vi "borrowDataDescriptorInterface.vi"(8 "error in (no error)":errorcluster, 11 "IBaseObject in":refnum<class "IBaseObject.lvclass">) -> (0 "error out":errorcluster, 2 "DataDescriptor out":refnum<class "IDataDescriptor.lvclass">, 3 "IBaseObject out":refnum<class "IBaseObject.lvclass">)   [LabVIEW 2022 SP3, in "openDAQ.lvlib" / "IBaseObject.lvlib" / "IBaseObject.lvclass"]
uses:
  <instrlib>/openDAQ/Public/Classes/IBaseObject/IBaseObject.lvclass
  <instrlib>/openDAQ/Public/Classes/IDataDescriptor/IDataDescriptor.lvclass
  C:/Program Files (x86)/National Instruments/LabVIEW 2022/instr.lib/openDAQ/Public/Classes/IBaseObject/IBaseObject.lvclass
  <instrlib>/openDAQ/Public/Classes/IBaseObject/IBaseObject.lvclass/IBaseObject.ctl
  <instrlib>/openDAQ/Public/Classes/IBaseObject/Accessor/Read reference.vi
  <instrlib>/openDAQ/Public/Classes/IBaseObject/Accessor/Write reference.vi
  <instrlib>/openDAQ/Binaries/Windows/x86/copendaq32.dll
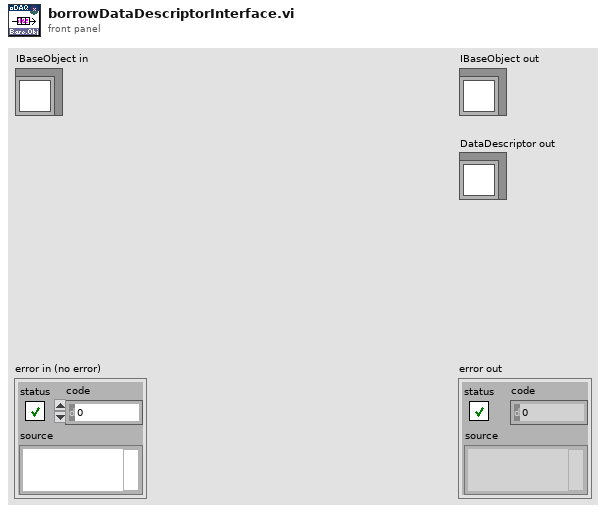
[diagram p1: front panel]
types:
  T1 = enum16{"big-endian, network order", "native, host order", "little-endian"}
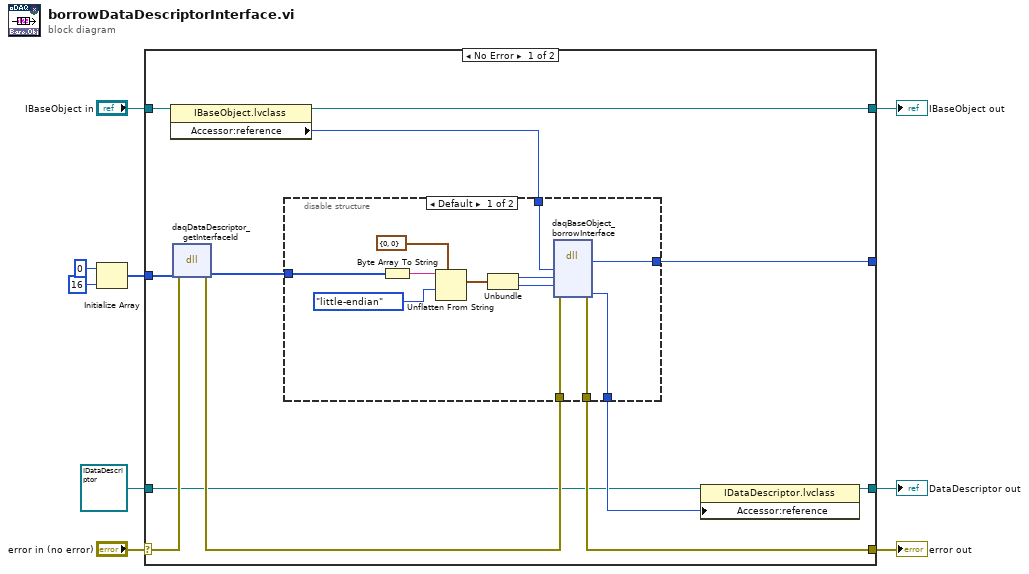
[diagram p0: block diagram]
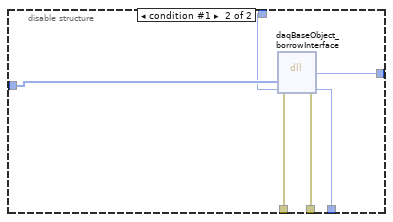
[diagram p2: hidden frame]
diagram:
  n1 = Initialize Array(u8 0, 16 ("dimension size")) -> (w1:u8[])
  n2 = case shown="No Error" "error in (no error)" {
    selector: "error in (no error)" -> [w18 w42]
    tunnel: [w20 w42] -> w8
    tunnel: [w11 w41] -> w6
    tunnel: "IBaseObject in" -> [w21 w41]
    tunnel: refnum<class "IDataDescriptor.lvclass"> refnum ("openDAQ.lvlib:IBaseObject.lvlib:IDataDescriptor.lvlib:IDataDescriptor.lvclass") -> [w12 w40]
    tunnel: w1 -> [w16 _]
    tunnel: [w14 w40] -> w4
    tunnel: [w10 _] -> _
    frame No Error {
      n3 = property class="IBaseObject.lvclass"(reference=w21) -> (reference out=w11:refnum<class "IBaseObject.lvclass">, "Accessor:reference"=w19:i64)  [unwired: 1 in, 1 out]
      n4 = dll-call lib="C:/Program Files (x86)/National Instruments/LabVIEW 2022/instr.lib/openDAQ/Binaries/Windows/x86/copendaq*.*" fn="daqDataDescriptor_getInterfaceId"(error in=w18, "id"=w16) -> (error out=w17:errorcluster, "id"=w13:u8[])  [unwired: 3 in, 1 out]
      n5 = disable-structure shown="Default" {
        disable-tunnel: [w33 w38] -> w20
        disable-tunnel: w19 -> [w23 w35]
        disable-tunnel: w17 -> [w32 w39]
        disable-tunnel: [w31 w37] -> w15
        disable-tunnel: w13 -> [w27 w36]
        disable-tunnel: [w22 w34] -> w10
        frame condition #0 (active) {
          n6 = Byte Array To String(unsigned byte array=w27) -> (string=w30:string)
          n7 = Unflatten From String(type=cluster{u64, u64} {0, 0}, binary string=w30, byte order (0:big-endian, network order)=T1."little-endian") -> (value=w28:cluster{u64, u64})  [unwired: 2 in, 2 out]
          n8 = Unbundle(w28) -> (w26:u64, w25:u64)
          n9 = dll-call lib="C:/Program Files (x86)/National Instruments/LabVIEW 2022/instr.lib/openDAQ/Binaries/Windows/x86/copendaq*.*" fn="daqBaseObject_borrowInterface"(error in=w32, "self"=w23, "intfId1"=w26, "intfId2"=w25) -> (error out=w33:errorcluster, "return type"=w22:u32, "interfacePtr"=w31:i64)  [unwired: 6 in, 1 out]
        }
        frame condition #1 {
          n10 = dll-call lib="C:/Program Files (x86)/National Instruments/LabVIEW 2022/instr.lib/openDAQ/Binaries/Windows/x86/copendaq*.*" fn="daqBaseObject_borrowInterface"(error in=w39, "intfId"=w36, "interfacePtr"=w35) -> (error out=w38:errorcluster, "return type"=w34:u32, "interfacePtr"=w37:i64)  [unwired: 3 in, 1 out]
        }
      }
      n11 = property class="IDataDescriptor.lvclass"(reference=w12, "Accessor:reference"=w15) -> (reference out=w14:refnum<class "IDataDescriptor.lvclass">)  [unwired: 1 in, 1 out]
    }
    frame Error {
    }
  }
  "error out" <- w8
  "IBaseObject out" <- w6
  "DataDescriptor out" <- w4
